vi "ReadHead.vi"(0 "new file path":path=path "C:/WINDOWS/DESKTOP/rri.eye") -> (4 "Compression Parameters":T1 {"duration" format="%#_3g"; "% taper" min=50 max=1000 format="%.2f"; "F2 (MHz)" format="%.3f"; "F1 (MHz)" format="%.3f"}, 5 "Therapy Parameters":T5 {"Therapy amplitude (mV)" min=50 max=1000 format="%.2f"; "Time on (s)" format="%.3f"; "Theraputic Freq (MHz)" format="%.3f"}, 6 "Header In":T3={"header info"={"Header"="", "Head length"=0}, "A/D info"={"# rf points per line"=0, "# lines per scan"=0, "sample rate MHz"=0, "# A/D bits"=0, "# bytes per A/D"=0, "TGC Flag"=0, "A/D Type"=""}, "Tranducer Info"={"bandwidth"=0.0, "center freq"=0.0, "start freq"=0.0, "ID"=0}, "Scan Info"={"delay"=0.0, "pivot distance"=0.0, "sector scan angle"=0.0, "operator"="", "Scan Mode"="", "location"=""}, "Time/Date Info"={"date"="", "time"=""}, "RF Info"={"RF file name"="", "RF file att"="", "RF cal file name"="", "RF cal file att"=""}, "Patient Info"={"ID"="", "extended ID"="", "age"=0, "sex"="", "previously\nscanned"="", "PSA"=0.0, "LOS"=1, "Ethnicty 2"=3, "Race"=3}, "Tissue Type"={"organ"=0, "disease type"=0, "disease location"=0, "IQ_pts"=0, "RcvBuffer"=0, "RcvFrame"=0, "IQBuff"=0, "IQFrame"=0, "IQPage"=0}, "Votage scaling"={"Digitizer (dB)"=0.0, "Gain (dB)"=0.0, "Atten (dB)"=0.0}, "Comment"="", "Misc Info"={"avg num"=0, "c speed"=0, "Div By or SF zones"=0, "XMIT CHS"=0, "RCV CHS"=0, "Xmit angle"=0.0}, "Therapy Parameters"={"Theraputic Freq (MHz)"=0.1, "Time on (s)"=1.0, "Therapy amplitude (mV)"=50.0, "Lines Before"=20, "Lines After"=80}, "Scan Settings"={"Energy (uJ or V)"=0, "Damp (Ohm) or Fc"=0, "HP Filt (KHz)"=0, "LP Filt (MHz)"=0, "Gain (db)"=0, "prf (kHz)"=0.0, "Distance between\nscan lines (um)"=0, "Distance between\nscan planes (um)"=0, "Scan line gap (um)"=0.0, "Scan plane gap (um)"=0.0}, "Compression Parameters"={"F1 (MHz)"=0.0, "F2 (MHz)"=0.0, "% taper"=0.0, "duration"=0.0}, "Patient Info Xtra"={"First Name"="", "Last Name"="", "Notes"=""}, "ROI Box"=[]} {"Compression Parameters"."% taper" min=50 max=1000 format="%.2f"; "Compression Parameters"."F2 (MHz)" format="%.3f"; "Compression Parameters"."F1 (MHz)" format="%.3f"; "Scan Settings"."prf (kHz)" format="%.2f"; "Therapy Parameters"."Therapy amplitude (mV)" min=50 max=1000 format="%.2f"; "Therapy Parameters"."Time on (s)" format="%.3f"; "Therapy Parameters"."Theraputic Freq (MHz)" format="%.3f"; "Patient Info"."Race" items=["Am Ind or Alaska", "Asian", "Hawaiian, Pac Isl", "Black or Afr Amer", "White", "more than one race", "unknown"]; "Patient Info"."Ethnicty 2" items=["Hispanic", "Non-Hispanic", "unknown"]; "Patient Info"."LOS" items=["1", "2", "3", "4", "5"]; "Patient Info"."PSA" format="%.1f"; "Scan Info"."delay" format="%.2f"; "Scan Info"."pivot distance" format="%.2f"; "Scan Info"."sector scan angle" format="%.2f"; "Tranducer Info"."bandwidth" format="%.2f"; "Tranducer Info"."center freq" format="%.2f"; "Tranducer Info"."start freq" format="%.2f"}, 7 "Pan Scan Settings":T4 {"prf (kHz)" format="%.2f"; "Gain (db)" items=["26.0", "40.0", "54.0"]; "LP Filt (MHz)" items=["20", "50", "100", "200"]; "HP Filt(KHz)" items=["1", "1000", "3000", "10000"]; "Damping (In Ohm)" items=["7", "10", "16", "20", "26", "30", "40", "50"]; "Energy (microJ)" items=["1", "2", "4", "8", "16", "32"]}, 8 "whole header":string, 9 "Comment":string, 10 "header info":cluster{"Header":string, "Head length":i16}, 11 "Misc Items":T7, 12 "A/D info":T13, 13 "Votage scaling":T8, 14 "Tranducer Info":T12 {"bandwidth" format="%.2f"; "center freq" format="%.2f"; "start freq" format="%.2f"}, 15 "Scan Info":T11 {"delay" format="%.2f"; "pivot distance" format="%.2f"; "sector scan angle" format="%.2f"}, 16 "Time/Date Info":cluster{"date":string, "time":string}, 17 "RF Info":T10={"RF file name"="", "RF file att"="", "RF cal file name"="impluse.cal", "RF cal file att"="0.0"}, 18 "Patient Info":T6={"ID"="", "extended ID"="", "age"=0, "sex"="", "previously\nscanned"="N", "PSA"=0.0, "LOS"=1, "Ethnicty 2"=3, "Ethnicty"=3} {"Ethnicty" items=["Am Ind or Alaska", "Asian", "Hawaiian, Pac Isl", "Black or Afr Amer", "White", "more than one race", "unknown"]; "Ethnicty 2" items=["Hispanic", "Non-Hispanic", "unknown"]; "LOS" items=["1", "2", "3", "4", "5"]; "PSA" format="%.1f"}, 19 "Tissue Type":T9)   [LabVIEW 2022 SP3]
uses:
  TimeDateInfo.vi
  ADInfo.vi
  Header.ctl
panel:
  out "WMC Scan Setting":T2={"Flag"=0, "Puls mode"=3, "Voltage [V]"=0, "Freq. [MHz]"=0, "Gain [dB]"=0, "not used"=0.0, "Distance between\nscan lines (mm)"=0, "Distance between\nscan planes (mm)"=0} {"Puls mode" items=["Half cycle positive", "Half cycle negegative", "Full cycle positive", "Full cycle negative"]; "not used" format="%.2f"}
  out "Ethnicty 3":u8(ring)=3 items=["Am Ind or Alaska", "Asian, Pac Islander", "Black, not Hispanic", "Hispanic", "White, not hispanic", "other, unknown"]
  # "Old style race indicator"
  # "© 2001 Riverside Research Institute"
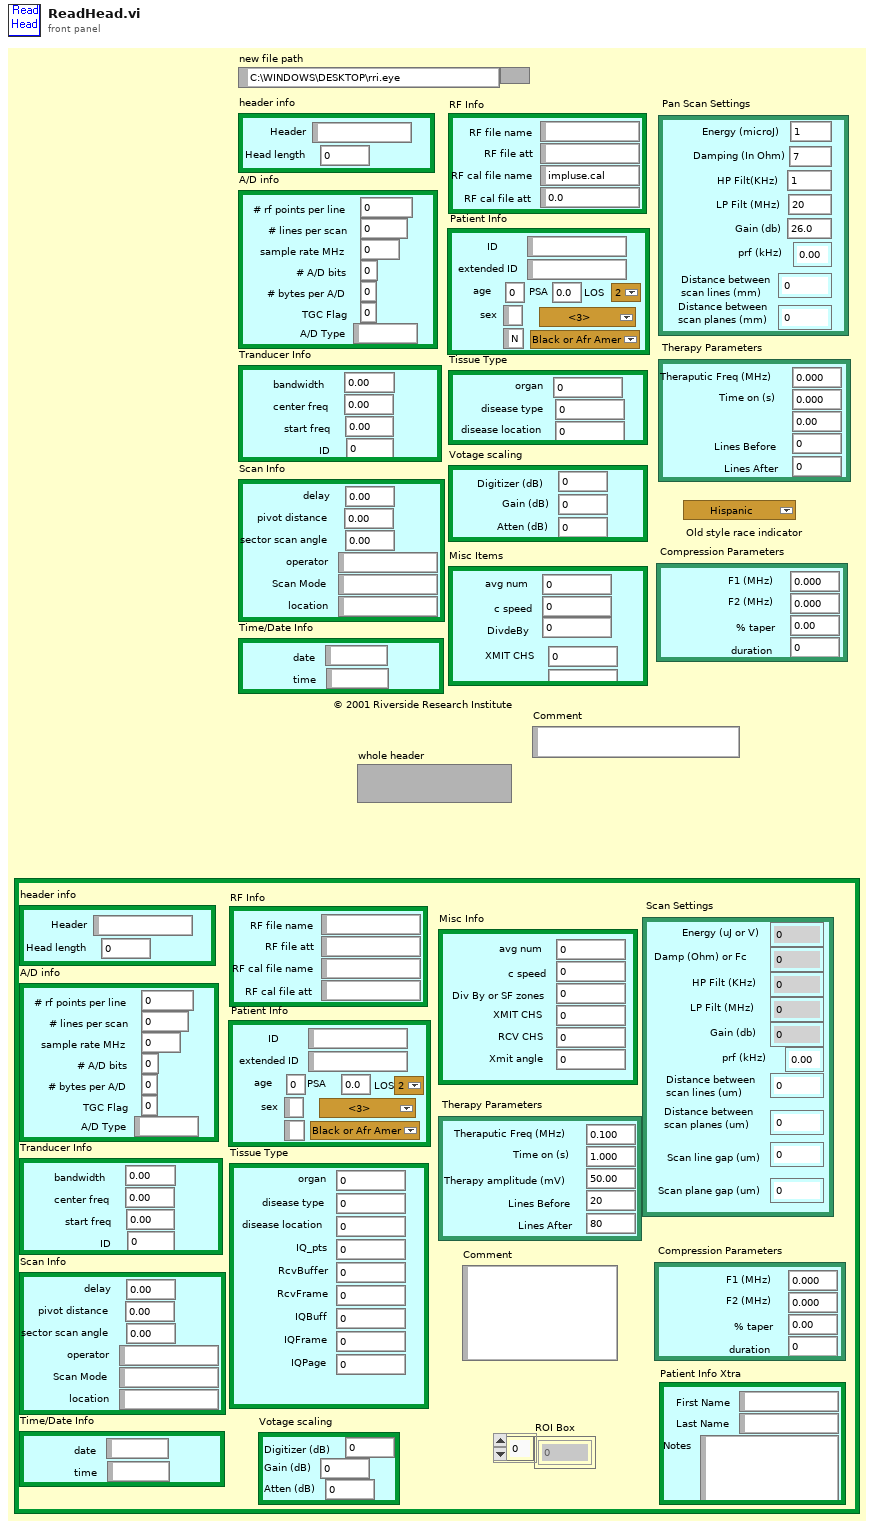
[diagram p1: front panel]
types:
  T1 = cluster{"F1 (MHz)":sgl, "F2 (MHz)":sgl, "% taper":sgl, "duration":sgl}
  T2 = cluster{"Flag":u8, "Puls mode":u16, "Voltage [V]":u8, "Freq. [MHz]":u8, "Gain [dB]":u8, "not used":sgl, "Distance between\nscan lines (mm)":u16, "Distance between\nscan planes (mm)":u16}
  T3 = typedef "Header.ctl" = cluster{"header info":cluster{"Header":string, "Head length":i16}, "A/D info":cluster{"# rf points per line":u16, "# lines per scan":u16, "sample rate MHz":u16, "# A/D bits":i16, "# bytes per A/D":u16, "TGC Flag":u16, "A/D Type":string}, "Tranducer Info":cluster{"bandwidth":sgl, "center freq":sgl, "start freq":sgl, "ID":i32}, "Scan Info":cluster{"delay":sgl, "pivot distance":sgl, "sector scan angle":sgl, "operator":string, "Scan Mode":string, "location":string}, "Time/Date Info":cluster{"date":string, "time":string}, "RF Info":cluster{"RF file name":string, "RF file att":string, "RF cal file name":string, "RF cal file att":string}, "Patient Info":cluster{"ID":string, "extended ID":string, "age":u16, "sex":string, "previously\nscanned":string, "PSA":sgl, "LOS":u8, "Ethnicty 2":u8, "Race":u8}, "Tissue Type":cluster{"organ":i16, "disease type":i16, "disease location":i16, "IQ_pts":u16, "RcvBuffer":u8, "RcvFrame":u16, "IQBuff":u8, "IQFrame":u16, "IQPage":u8}, "Votage scaling":cluster{"Digitizer (dB)":sgl, "Gain (dB)":sgl, "Atten (dB)":sgl}, "Comment":string, "Misc Info":cluster{"avg num":u16, "c speed":i16, "Div By or SF zones":i16, "XMIT CHS":u8, "RCV CHS":u8, "Xmit angle":sgl}, "Therapy Parameters":cluster{"Theraputic Freq (MHz)":sgl, "Time on (s)":sgl, "Therapy amplitude (mV)":sgl, "Lines Before":u16, "Lines After":u16}, "Scan Settings":cluster{"Energy (uJ or V)":u8, "Damp (Ohm) or Fc":u8, "HP Filt (KHz)":u8, "LP Filt (MHz)":u8, "Gain (db)":u8, "prf (kHz)":sgl, "Distance between\nscan lines (um)":u16, "Distance between\nscan planes (um)":u16, "Scan line gap (um)":sgl, "Scan plane gap (um)":sgl}, "Compression Parameters":cluster{"F1 (MHz)":sgl, "F2 (MHz)":sgl, "% taper":sgl, "duration":sgl}, "Patient Info Xtra":cluster{"First Name":string, "Last Name":string, "Notes":string}, "ROI Box":u16[]}
  T4 = cluster{"Energy (microJ)":u8, "Damping (In Ohm)":u8, "HP Filt(KHz) ":u8, "LP Filt (MHz)":u8, "Gain (db)":u8, "prf (kHz)":sgl, "Distance between\nscan lines (mm)":u16, "Distance between\nscan planes (mm)":u16}
  T5 = cluster{"Theraputic Freq (MHz)":sgl, "Time on (s)":sgl, "Therapy amplitude (mV)":sgl, "Lines Before":u16, "Lines After":u16}
  T6 = cluster{"ID":string, "extended ID":string, "age":u16, "sex":string, "previously\nscanned":string, "PSA":sgl, "LOS":u8, "Ethnicty 2":u8, "Ethnicty":u8}
  T7 = cluster{"avg num":i16, "c speed":i16, "DivdeBy":i16, "XMIT CHS":u8, "RCV CHS":u8}
  T8 = cluster{"Digitizer (dB)":sgl, "Gain (dB)":sgl, "Atten (dB)":sgl}
  T9 = cluster{"organ":i16, "disease type":i16, "disease location":i16}
  T10 = cluster{"RF file name":string, "RF file att":string, "RF cal file name":string, "RF cal file att":string}
  T11 = cluster{"delay":sgl, "pivot distance":sgl, "sector scan angle":sgl, "operator":string, "Scan Mode":string, "location":string}
  T12 = cluster{"bandwidth":sgl, "center freq":sgl, "start freq":sgl, "ID":i32}
  T13 = cluster{"# rf points per line":u16, "# lines per scan":u16, "sample rate MHz":u16, "# A/D bits":u16, "# bytes per A/D":u16, "TGC Flag":u16, "A/D Type":string}
  T14 = cluster{"# rf points per line":u16, "# lines per scan":u16, "sample rate MHz":u16, "# A/D bits":i16, "# bytes per A/D":u16, "TGC Flag":u16, "A/D Type":string}
  T15 = cluster{"ID":string, "Extended ID":string, "age":u16, "gender":string, "previously\nscanned":string, "PSA":sgl, "LOS":u8, "Ethnicty 3":u8, "Ethnicty 4":u8}
  T16 = cluster{"atten":i16, "cal sens":i16, "DivideBy":i16, "XMIT CHS":u8, "RCV CHS":u8}
  T17 = cluster{"ENERGY(UJ)":u8, "DAMPING (IN Ohm)":u8, "HP FILT(IN KHz) ":u8, "LP FILT(IN MHz)":u8, "GAIN(db)":u8, "prf (kHz)":sgl, "Distance between\nscan lines (mm)":u16, "Distance between\nscan planes (mm)":u16}
  T18 = cluster{"header info":cluster{"Header":string, "Head length":i16}, "A/D info":cluster{"# rf points per line":u16, "# lines per scan":u16, "sample rate MHz":u16, "# A/D bits":i16, "# bytes per A/D":u16, "TGC Flag":u16, "A/D Type":string}, "Tranducer Info":cluster{"bandwidth":sgl, "center freq":sgl, "start freq":sgl, "ID":i32}, "Scan Info":cluster{"delay":sgl, "pivot distance":sgl, "sector scan angle":sgl, "operator":string, "Scan Mode":string, "location":string}, "Time/Date Info":cluster{"date":string, "time":string}, "RF Info":cluster{"RF file name":string, "RF file att":string, "RF cal file name":string, "RF cal file att":string}, "Patient Info":cluster{"ID":string, "Extended ID":string, "age":u16, "gender":string, "previously\nscanned":string, "PSA":sgl, "LOS":u8, "Ethnicty 3":u8, "Ethnicty 4":u8}, "Tissue Type":cluster{"organ":i16, "disease type":i16, "disease location":i16}, "Votage scaling":cluster{"Digitizer (dB)":sgl, "Gain (dB)":sgl, "Atten (dB)":sgl}, "comment":string, "TGC & RF/AD Info":cluster{"atten":i16, "cal sens":i16, "DivideBy":i16, "XMIT CHS":u8, "RCV CHS":u8}, "Therapy Parameters":cluster{"Theraputic Freq (MHz)":sgl, "Time on (s)":sgl, "Therapy amplitude (mV)":sgl, "Lines Before":u16, "Lines After":u16}, "Scan Settings":cluster{"ENERGY(UJ)":u8, "DAMPING (IN Ohm)":u8, "HP FILT(IN KHz) ":u8, "LP FILT(IN MHz)":u8, "GAIN(db)":u8, "prf (kHz)":sgl, "Distance between\nscan lines (mm)":u16, "Distance between\nscan planes (mm)":u16}, "Compression Parameters":cluster{"F1 (MHz)":sgl, "F2 (MHz)":sgl, "% taper":sgl, "duration":sgl}, cluster{string, string, string}, "ROI Box":u16[]}
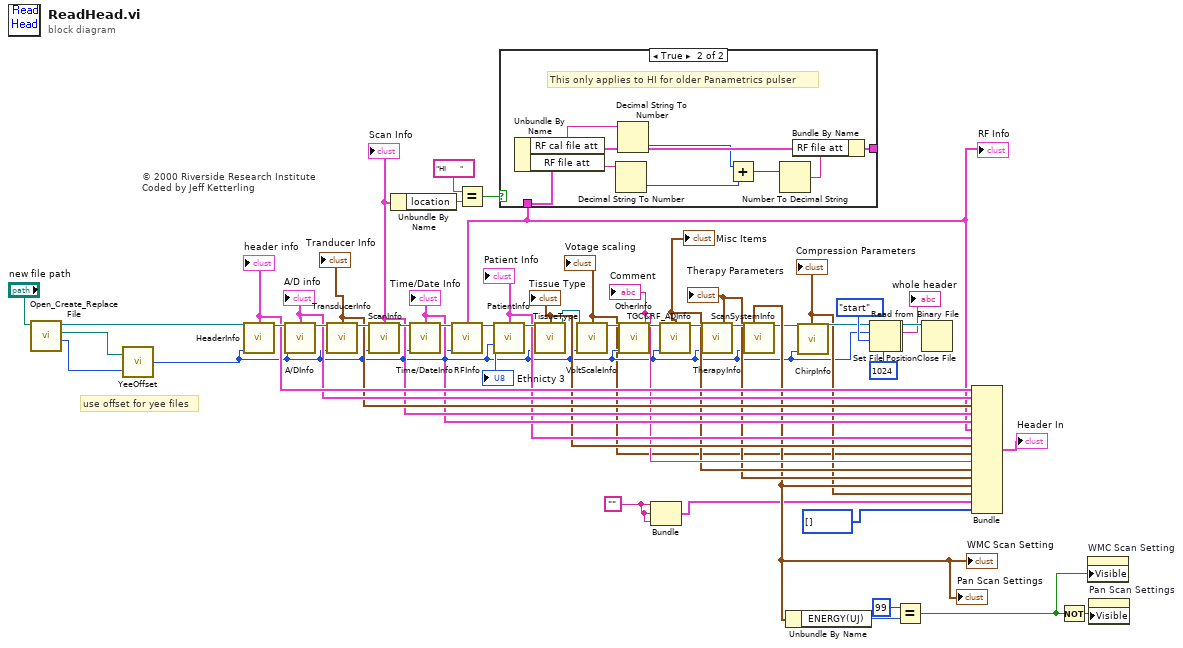
[diagram p0: block diagram]
diagram:
  w3 = ""
  # "use offset for yee files"
  # "© 2000 Riverside Research Institute\nCoded by Jeff Ketterling"
  n1 = call <vilib>:"Open_Create_Replace File.vi"("file path"="new file path") -> ("file size (bytes)"=w20:i32, "new file path"=w19:path, "refnum"=w22:refnum<file>)  [unwired: 5 in, 3 out]
  n2 = call "YeeOffset.vi"("file size (bytes)"=w20, "new file path"=w19) -> ("Numeric"=w5:i32)
  n3 = call "HeaderInfo.vi"("refnum"=w22, "offset"=w5) -> ("header info"=w34:cluster{"Header":string, "Head length":i16}, "dup refnum"=w47:refnum<file>)  [unwired: 12 out]
  "header info" <- w34
  n4 = call "A/DInfo.vi"("refnum"=w47, "offset"=w5) -> ("A/D info"=w33:T14, "dup refnum"=w46:refnum<file>)  [unwired: 12 out]
  "A/D info" <- w33
  n5 = call "TransducerInfo.vi"("refnum"=w46, "offset"=w5) -> ("Tranducer Info"=w32:T12, "dup refnum"=w45:refnum<file>)  [unwired: 12 out]
  "Tranducer Info" <- w32
  n6 = call "ScanInfo.vi"("refnum"=w45, "offset"=w5) -> ("Scan Info"=w31:T11, "dup refnum"=w44:refnum<file>)  [unwired: 12 out]
  "Scan Info" <- w31
  n7 = Unbundle By Name(w31) -> ("location"=w37:string)
  n8 = call "Time/DateInfo.vi"("refnum"=w44, "offset"=w5) -> ("Time/Date Info"=w30:cluster{"date":string, "time":string}, "dup refnum"=w43:refnum<file>)  [unwired: 12 out]
  "Time/Date Info" <- w30
  n9 = call "RFInfo.vi"("refnum"=w43, "offset"=w5) -> ("RF Info"=w8:T10, "dup refnum"=w42:refnum<file>)  [unwired: 12 out]
  "RF Info" <- w8
  n10 = Equal?(x="HI       ", y=w37) -> (x = y?=w35:bool)
  n11 = call "PatientInfo.vi"("refnum"=w42, "offset"=w5) -> ("Patient Info"=w29:T15, "dup refnum"=w41:refnum<file>, "Ethnicity"=→"Ethnicty 3":u8)  [unwired: 11 out]
  "Patient Info" <- w29
  n12 = case shown="True" w35 {
    tunnel: w8 -> [w52 w57]
    tunnel: [w52 w55] -> _
    frame False {
    }
    frame True {
      # "This only applies to HI for older Panametrics pulser"
      n13 = Unbundle By Name(w57) -> ("RF cal file att"=w54:string, "RF file att"=w60:string)
      n14 = Decimal String To Number(string=w60) -> (number=w59:i32)  [unwired: 3 out]
      n15 = Decimal String To Number(string=w54) -> (number=w53:i32)  [unwired: 3 out]
      n16 = Add(x=w53, y=w59) -> (x+y=w58:i32)
      n17 = Number To Decimal String(number=w58) -> (decimal integer string=w56:string)  [unwired: 1 out]
      n18 = Bundle By Name(cluster=w57, "RF file att"=w56) -> (w55:T10)
    }
  }
  n19 = call "TissueType.vi"("refnum"=w41, "offset"=w5) -> ("Tissue Type"=w28:T9, "dup refnum"=w7:refnum<file>)  [unwired: 12 out]
  "Tissue Type" <- w28
  n20 = call "VoltScaleInfo.vi"("refnum"=w7, "offset"=w5) -> ("Votage scaling"=w4:T8, "dup refnum"=w6:refnum<file>)  [unwired: 12 out]
  "Votage scaling" <- w4
  n21 = call "OtherInfo.vi"("refnum"=w6, "offset"=w5) -> ("dup refnum"=w40:refnum<file>, "comment"=w27:string)  [unwired: 12 out]
  "Comment" <- w27
  n22 = Bundle(w3, w3, w3) -> (w2:cluster{string, string, string})  [unwired: 1 in]
  n23 = call "TGC&RF_ADInfo.vi"("refnum"=w40, "offset"=w5) -> ("TGC & RF/AD Info"=w26:T16, "dup refnum"=w39:refnum<file>)  [unwired: 12 out]
  "Misc Items" <- w26
  n24 = call "TherapyInfo.vi"("refnum"=w39, "offset"=w5) -> ("Therapy Parameters"=w25:T5, "dup refnum"=w38:refnum<file>)  [unwired: 12 out]
  "Therapy Parameters" <- w25
  n25 = call "ScanSystemInfo.vi"("refnum"=w38, "offset"=w5) -> ("Scan Settings"=w14:T17, "dup refnum"=w10:refnum<file>)  [unwired: 12 out]
  "Pan Scan Settings" <- w14
  "WMC Scan Setting" <- w14
  n26 = Unbundle By Name(w14) -> ("ENERGY(UJ)"=w17:u8)
  n27 = call "ChirpInfo.vi"("offset"=w5, "refnum"=w10) -> ("refnum out"=w11:refnum<file>, "Compression Parameters"=w9:T1)  [unwired: 8 out]
  "Compression Parameters" <- w9
  n28 = Set File Position(offset (in bytes) (0)=w5, refnum=w11, from (0:start)=enum16{"start", "end", "current"}."start" ("pos mode (0:2)")) -> (refnum out=w13:refnum<file>, error out=w12:errorcluster)  [unwired: 1 in]
  n29 = Read from Binary File(8:w12, 10:1024 ("count"), 11:w13) -> (2:→"whole header":string, 3:w49:refnum<file>)  [unwired: 5 out]
  n30 = Equal?(x=99, y=w17) -> (x = y?=w16:bool)
  n31 = Close File(refnum=w49) -> ()  [unwired: 1 in, 2 out]
  n32 = Bundle("header info"=w34, "A/D info"=w33, "Tranducer Info"=w32, "Scan Info"=w31, "Time/Date Info"=w30, "RF Info"=w8, "Patient Info"=w29, "Tissue Type"=w28, "Votage scaling"=w4, "comment"=w27, "TGC & RF/AD Info"=w26, "Therapy Parameters"=w25, "Scan Settings"=w14, "Compression Parameters"=w9, w2, "ROI Box"=u16[] []) -> (→"Header In":T18)  [unwired: 1 out]
  n33 = Not(x=w16) -> (.not. x?=w15:bool)
  n34 = property on="WMC Scan Setting" class="Clust (strict)"("Visible"=w16) -> ()  [unwired: 2 in, 2 out]
  n35 = property on="Pan Scan Settings" class="Clust (strict)"("Visible"=w15) -> ()  [unwired: 2 in, 2 out]
